vi "Beta 1.vi"() -> ()   [LabVIEW 2012]
uses:
  Arc/Alt Control.ctl
  Type Defs/Single Digit 3.ctl
panel:
  in  "stop":bool
  in  "Tab Control":T1(tab)
  out "Altitude Message":string
  out "Altittude":T2={"Single Digit 4"=9, "Single Digit 4"=9, "Single Digit 5"=9, "Single Digit 6"=9, "Single Digit 7"=9} {"Single Digit 7" min=0 max=9 step=1 format="%1.0g"; "Single Digit 6" min=0 max=9 step=1 format="%1.0g"; "Single Digit 5" min=0 max=9 step=1 format="%1.0g"; "Single Digit 4" min=0 max=9 step=1 format="%1.0g"; "Single Digit 4" min=0 max=9 step=1 format="%1.0g"}
  in  "Mode":cluster{"Run":bool, "Hold":bool, "Off":bool}
  out "Temp C":dbl=1001.8
  out "Press mB":dbl=1001.8
  in  "System Status":cluster{bool, bool, bool, bool, bool, bool}={TRUE, TRUE, TRUE, TRUE, TRUE, TRUE}
  out "Time Stamp":timestamp
  out "Altitude 3":dbl=88890.0
  in  "Confirm Now":bool
  in  "Notes":string
  in  "Datlog File":path
  out "Waveform Graph 2":dbl[](graph)
  out "Waveform Graph":dbl[](graph)
  in  "Altitude 2":dbl=88890.0
  out "Altitude":dbl=88888.0
  # "Current Effective Altitude in  Meters"
  # "M\ne\nt\ne\nr\ns"
  # "WARNING"
  # "%"
  # "CO2"
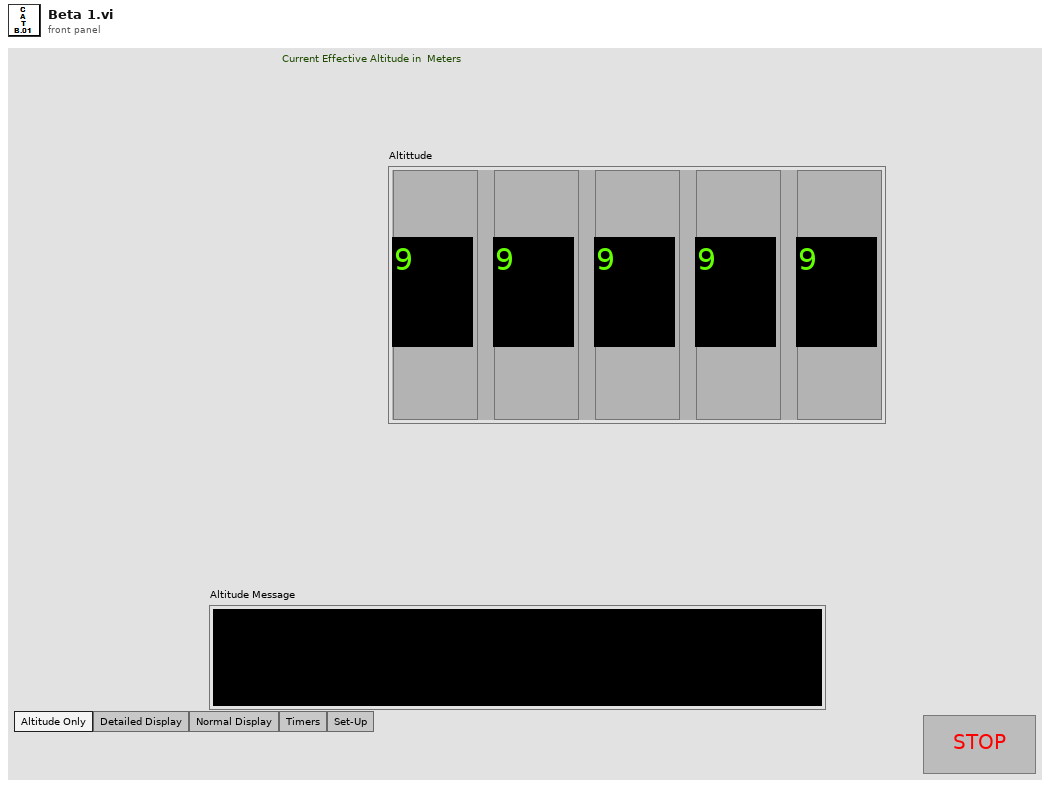
[diagram p1: front panel]
types:
  T1 = enum32{"Altitude Only", "Detailed Display", "Normal Display", "Timers", "Set-Up"}
  T2 = typedef "Alt Control.ctl" = cluster{"Single Digit 4":T3, "Single Digit 4":T3, "Single Digit 5":T3, "Single Digit 6":T3, "Single Digit 7":T3}
  T3 = typedef "Single Digit 3.ctl" = i8
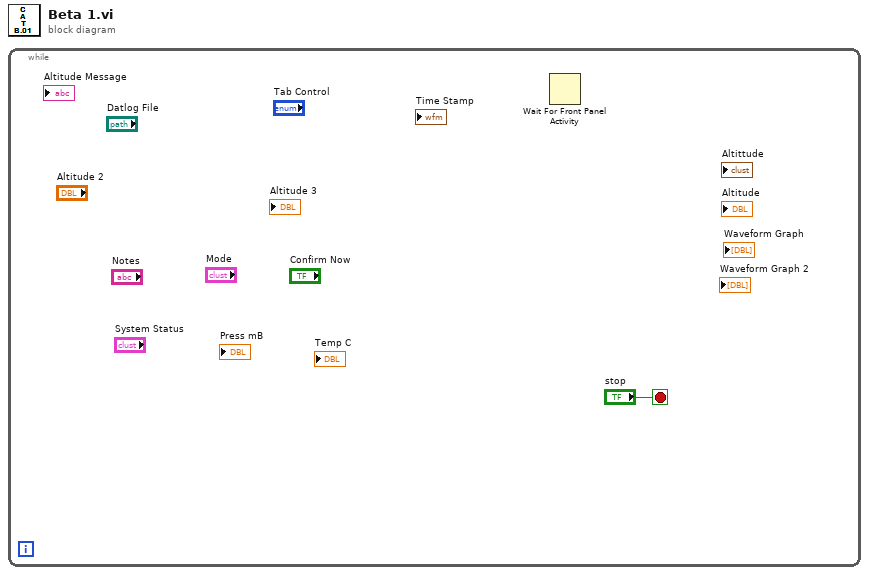
[diagram p0: block diagram]
diagram:
  n1 = while {
    stop <- "stop" stop-if-true
    n2 = Wait For Front Panel Activity() -> ()  [unwired: 3 in, 1 out]
  }
